vi "CDW_SpecPage.vi"(10 "Spec Page Interface":T2, 11 "MetaDataObj in":refnum<class "MetaDataObj.lvclass">) -> (3 "MetaDataObj out":refnum<class "MetaDataObj.lvclass">)   [LabVIEW 2019, in "NIVS_Consolidated_CDW_MetaDataObj.lvclass"]
uses:
  NIVS_Consolidated_CDW_MetaDataObj.lvclass
  Execution Mode.ctl
  Template Classes/NIVS_Asynchronous/NIVS_Asynchronous.lvclass
  Template Classes/NIVS_Inline HW Interface (Inline-Async)/NIVS_Inline HW Interface (Inline-Async).lvclass
  Template Classes/NIVS_Inline HW Interface/NIVS_Inline HW Interface.lvclass
  Template Classes/NIVS_Inline Model Interface/NIVS_Inline Model Interface.lvclass
  Template Classes/NIVS_Inline Timing and Sync/NIVS_Inline Timing and Sync.lvclass
  Template Classes/NIVS_Asynchronous Timing and Sync/NIVS_Asynchronous Timing and Sync.lvclass
  C:/Program Files (x86)/National Instruments/LabVIEW 2019/resource/dialog/NewProjectWizard/MetaDataObj/MetaDataObj.lvclass
  Template Classes/NIVS_CD Template/NIVS_CD Template.lvclass
  Template Classes/NIVS_PPL_Inline HW Interface (Inline-Async)/NIVS_PPL_Inline HW Interface (Inline-Async).lvclass
  C:/Users/nitest/Git/LabVIEW CD Template Fork/ProjectTemplate/Source/NI VeriStand/Custom Device/Template Classes/NIVS_CD Template/NIVS_CD Template.lvclass
  C:/Users/nitest/Git/LabVIEW CD Template Fork/ProjectTemplate/Source/NI VeriStand/Custom Device/Template Classes/NIVS_Timing and Sync (Abstract)/NIVS_Timing and Sync (Abstract).lvclass
  <resource>/dialog/NewProjectWizard/Spec Page Interface.ctl
  <resource>/dialog/NewProjectWizard/MetaDataObj/MetaDataObj.lvclass
panel:
  in  "PPL Build":bool=TRUE
  in  "Inline-Async":bool=TRUE
  in  "Custom Device Execution Mode":T1(ring)=enum."Inline HW Interface"
  in  "Custom Device Name":string
  in  "Project Root":path
  in  "Maximum Custom Device Instances":u32=1 min=1 max=2474 step=1
  in  "Insert Custom Device in submenu":bool
  in  "Parent Menu Name":string
  in  "Custom Device Extra Page Names":string[](array[string])
  # "Advanced Options"
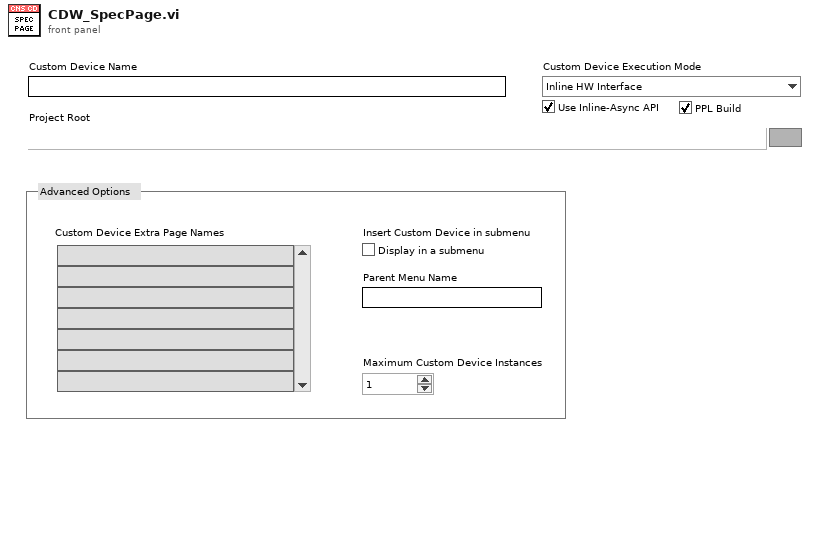
[diagram p1: front panel]
types:
  T1 = enum16{"Asynchronous", "Inline HW Interface", "Inline Model Interface", "Inline Timing and Sync", "Asynchronous Timing and Sync"}
  T2 = typedef "Spec Page Interface.ctl" = cluster{"\"Tab Forward To\" Refnum":refnum<vi>, "\"Tab Backward To\" Refnum":refnum<vi>, "Errors":refnum<user-event>, "Quit":refnum<user-event>}
  T3 = enum8{"Enabled", "Disabled", "Disabled and Grayed Out"}
  T4 = typedef "NIVS_Consolidated_CDW_MetaDataObj.lvclass/Execution Mode.ctl" = enum16{"Asynchronous", "Inline HW Interface", "Inline Model Interface", "Inline Timing and Sync", "Asynchronous Timing and Sync"}
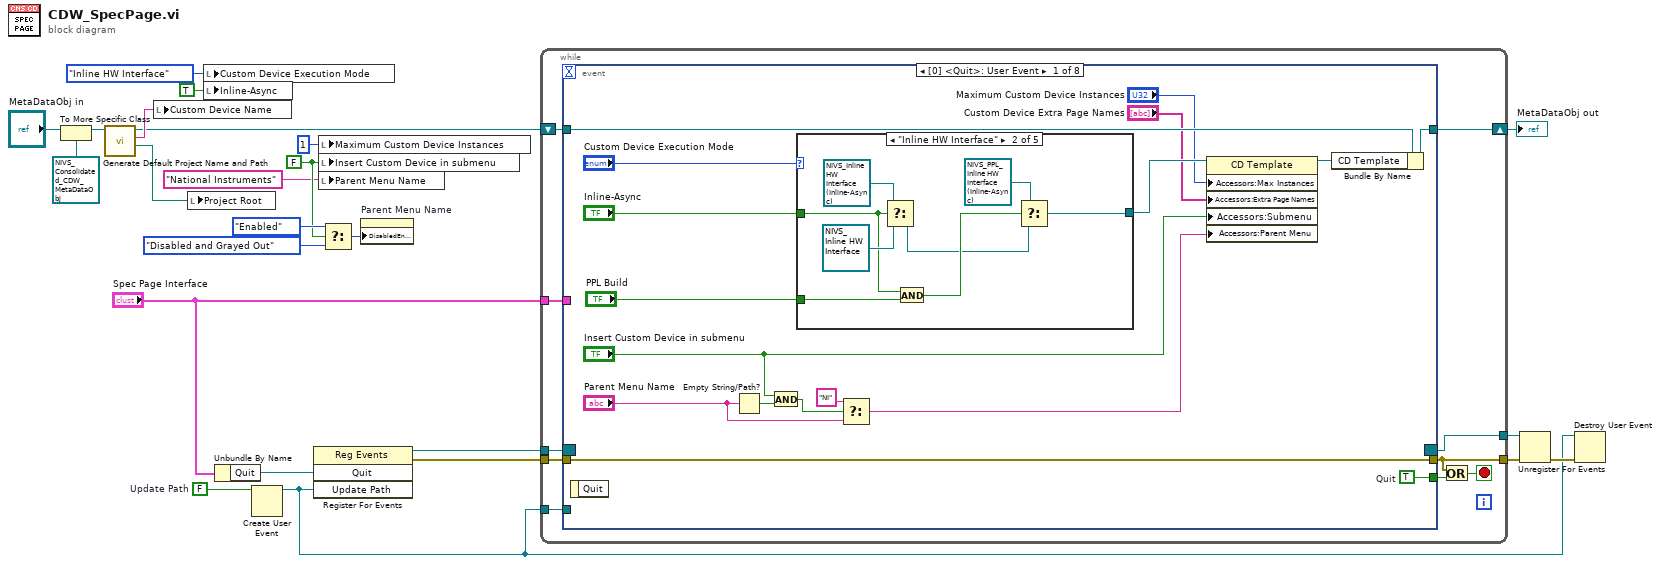
[diagram p0: block diagram]
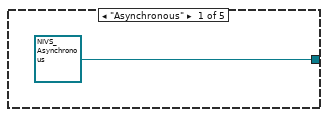
[diagram p2: hidden frame]
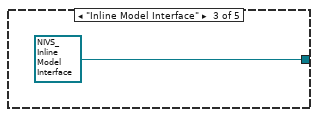
[diagram p3: hidden frame]
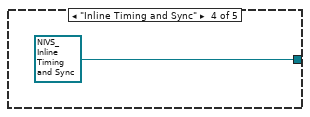
[diagram p4: hidden frame]
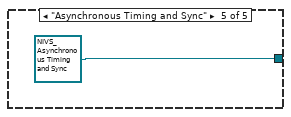
[diagram p5: hidden frame]
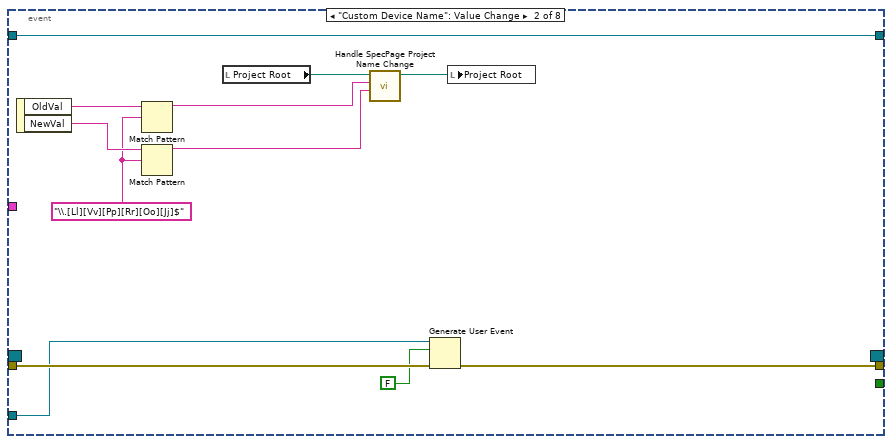
[diagram p6: hidden frame]
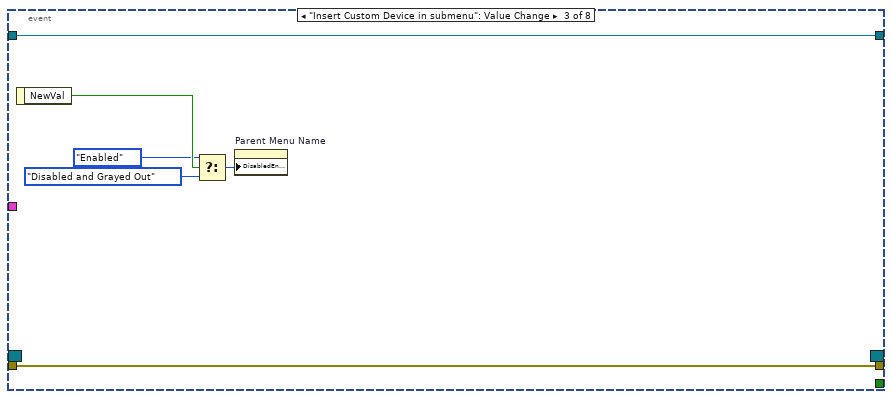
[diagram p7: hidden frame]
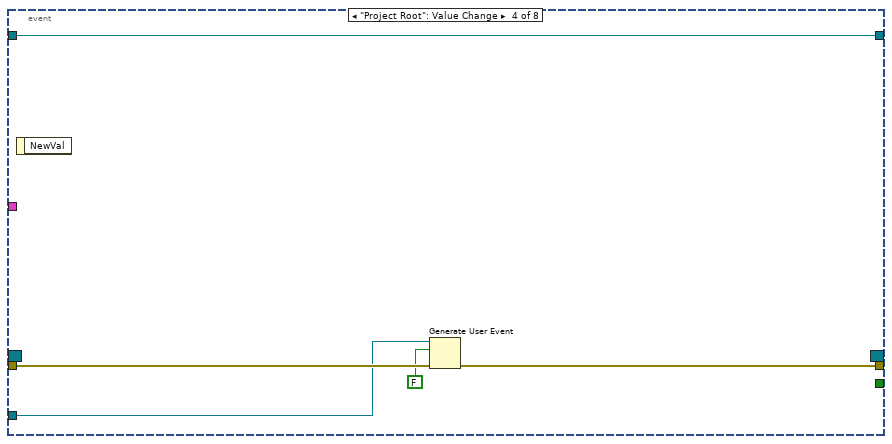
[diagram p8: hidden frame]
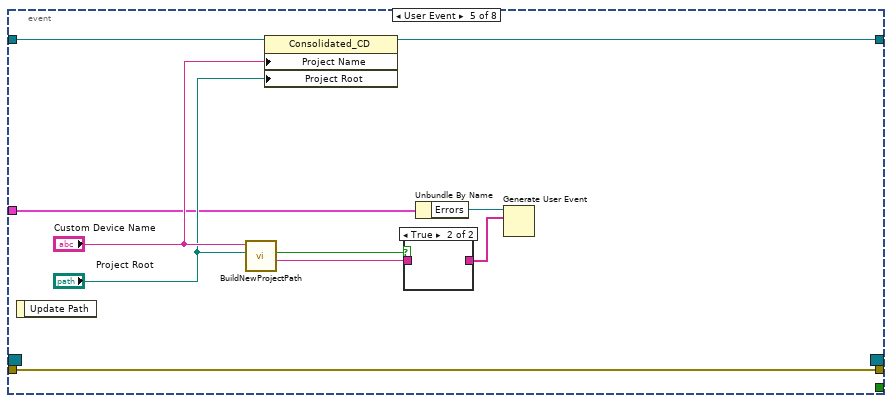
[diagram p9: hidden frame]
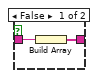
[diagram p10: hidden frame]
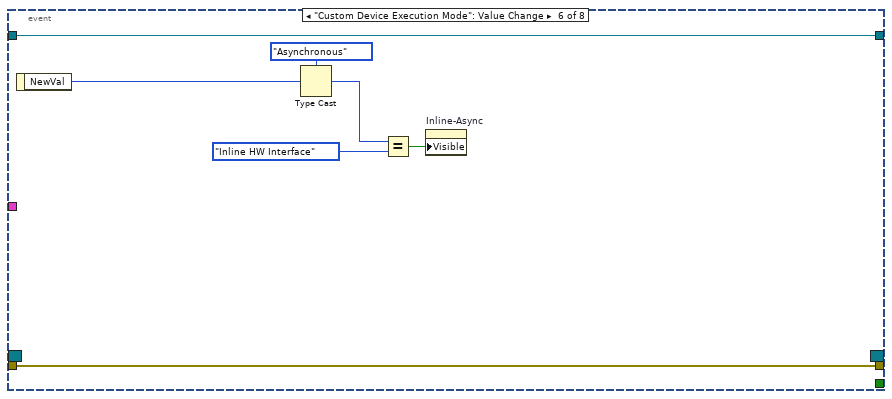
[diagram p11: hidden frame]
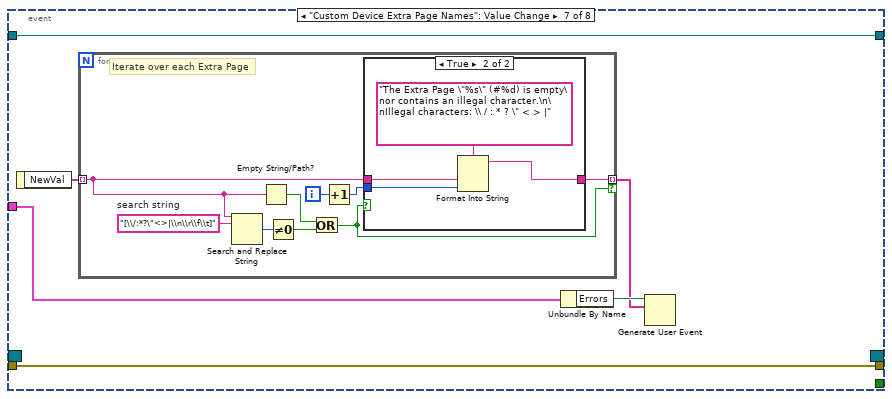
[diagram p12: hidden frame]
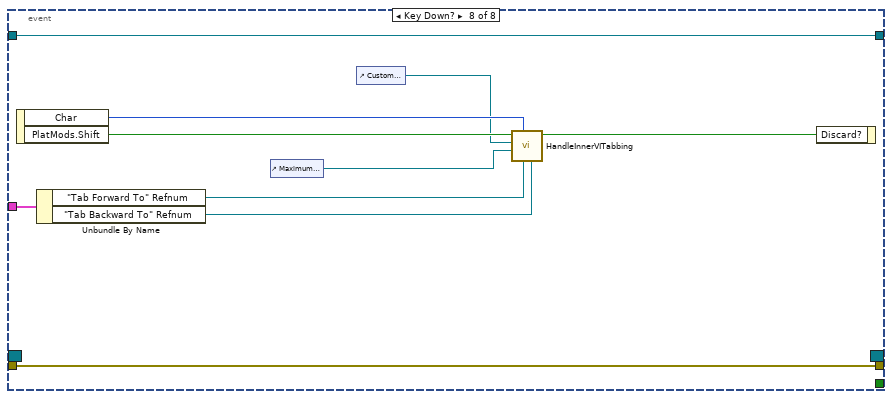
[diagram p14: hidden frame]
diagram:
  w5 = FALSE
  w8 = FALSE  # Update Path
  n1 = To More Specific Class(target class=refnum<class "NIVS_Consolidated_CDW_MetaDataObj.lvclass"> refnum ("Consolidated"), reference="MetaDataObj in") -> (specific class reference=w11:refnum<class "NIVS_Consolidated_CDW_MetaDataObj.lvclass">)  [unwired: 1 in, 1 out]
  n2 = call <resource>:"Generate Default Project Name and Path.vi"("DNL_MetaDataObj in"=w11) -> ("Project Root"=w9:path, "Project Name"=w14:string, "DNL_MetaDataObj out"=w10:refnum<class "NIVS_Consolidated_CDW_MetaDataObj.lvclass">)  [unwired: 8 in]
  n3 = local write "Custom Device Name"(w14) -> ()
  n4 = local write "Project Root"(w9) -> ()
  n5 = local write "Custom Device Execution Mode"(T1."Inline HW Interface" ("Custom Device Execution Mode")) -> ()
  n6 = local write "Inline-Async"(TRUE ("Inline-Async")) -> ()
  n7 = Unbundle By Name("Spec Page Interface") -> ("Quit"=w24:refnum<user-event>)
  n8 = Create User Event(user event datatype=w8) -> (user event=w6:refnum<user-event>)  [unwired: 1 in, 1 out]
  n9 = register-events(w24, w6) -> (reference out=w23:refnum<event-registration>, error out=w19:errorcluster)  [unwired: 2 in]
  n10 = local write "Maximum Custom Device Instances"(u32 1 ("Maximum Custom Device Instances")) -> ()
  n11 = local write "Insert Custom Device in submenu"(w5) -> ()
  n12 = local write "Parent Menu Name"("National Instruments") -> ()
  n13 = Select(t=T3."Enabled" ("Disabled"), s=w5, f=T3."Disabled and Grayed Out") -> (s? t:f=w17:T3)
  n14 = property on="Parent Menu Name" class="Str"("DisabledEnum"=w17) -> ()  [unwired: 2 in, 2 out]
  n15 = while {
    tunnel: "Spec Page Interface" -> [w32]
    shift-right: [w31] -> w20
    shift-left: w10 -> [w30]
    tunnel: w23 -> [w34]
    tunnel: w19 -> [w33]
    tunnel: [w27] -> w21
    tunnel: [w26] -> w13
    tunnel: w6 -> [w25]
    stop <- w29 stop-if-true
    n16 = event shown="[0] <Quit>: User Event" {
      selector: w34 -> [_ _ _ _ _ _ _ _]
      dyn-events: [_ _ _ _ _ _ _ _] -> w26
      timeout: _ -> [_ _ _ _ _ _ _ _]
      tunnel: w32 -> [_ _ _ _ w91 _ w107 w130]
      tunnel: [w51 _ _ _ _ _ _ _] -> w28
      tunnel: [w50 w66 w81 w84 w96 w105 w111 w135] -> w27
      tunnel: w33 -> [w50 w75 w81 w86 w96 w105 w111 w135]
      tunnel: [w48 w74 w80 w85 w94 w104 w109 w134] -> w31
      tunnel: w30 -> [w49 w74 w80 w85 w95 w104 w109 w134]
      tunnel: w25 -> [_ w65 _ w83 _ _ _ _]
      event User Event {
        w51 = TRUE  # Quit
        n17 = event-data() -> ()  [unwired: 1 in, 1 out]
        n18 = Empty String/Path?(string/path="Parent Menu Name") -> (empty?=w46:bool)
        n19 = And(x="Insert Custom Device in submenu", y=w46) -> (x .and. y?=w45:bool)
        n20 = case shown="\"Inline HW Interface\"" "Custom Device Execution Mode" {
          tunnel: "Inline-Async" -> [_ w57 _ _ _]
          tunnel: [refnum<class "NIVS_Asynchronous.lvclass"> refnum ("NIVS_Asynchronous.lvclass") w53 refnum<class "NIVS_Inline Model Interface.lvclass"> refnum ("NIVS_Inline Model Interface.lvclass") refnum<class "NIVS_Inline Timing and Sync.lvclass"> refnum ("NIVS_Inline Timing and Sync.lvclass") refnum<class "NIVS_Asynchronous Timing and Sync.lvclass"> refnum ("NIVS_Asynchronous Timing and Sync.lvclass")] -> w40
          tunnel: "PPL Build" -> [_ w58 _ _ _]
          frame "Asynchronous" {
          }
          frame "Inline HW Interface" {
            n21 = Select(t=refnum<class "NIVS_Inline HW Interface (Inline-Async).lvclass"> refnum ("NIVS_Inline HW Interface (Inline-Async).lvclass"), s=w57, f=refnum<class "NIVS_Inline HW Interface.lvclass"> refnum ("NIVS_Inline HW Interface.lvclass")) -> (s? t:f=w55:refnum<class "NIVS_CD Template.lvclass">)
            n22 = And(x=w57, y=w58) -> (x .and. y?=w56:bool)
            n23 = Select(t=refnum<class "NIVS_PPL_Inline HW Interface (Inline-Async).lvclass"> refnum ("NIVS_PPL_Inline HW Interface (Inline-Async).lvclass"), s=w56, f=w55) -> (s? t:f=w53:refnum<class "NIVS_CD Template.lvclass">)
          }
          frame "Inline Model Interface" {
          }
          frame "Inline Timing and Sync" {
          }
          frame "Asynchronous Timing and Sync" {
          }
        }
        n24 = Select(t="NI", s=w45, f="Parent Menu Name") -> (s? t:f=w36:string)
        n25 = property class="CD Template"(reference=w40, "Accessors:Max Instances"="Maximum Custom Device Instances", "Accessors:Extra Page Names"="Custom Device Extra Page Names", "Accessors:Submenu"="Insert Custom Device in submenu", "Accessors:Parent Menu"=w36) -> (reference out=w41:refnum<class "NIVS_CD Template.lvclass">)  [unwired: 1 in, 1 out]
        n26 = Bundle By Name(cluster=w49, "CD Template"=w41) -> (w48:refnum<class "NIVS_Consolidated_CDW_MetaDataObj.lvclass">)
      }
      event "Custom Device Name": Value Change {
        w71 = "\\.[Ll][Vv][Pp][Rr][Oo][Jj]$"
        n27 = event-data() -> ("OldVal"=w73:string, "NewVal"=w72:string)  [unwired: 1 in]
        n28 = Match Pattern(string=w73, regular expression=w71) -> (before substring=w68:string)  [unwired: 1 in, 3 out]
        n29 = Match Pattern(string=w72, regular expression=w71) -> (before substring=w67:string)  [unwired: 1 in, 3 out]
        n30 = local read "Project Root"() -> (w70:path)
        n31 = call <resource>:"Handle SpecPage Project Name Change.vi"("Project Name New Value"=w67, "Project Name Old Value"=w68, "Project Root in"=w70) -> ("Project Root out"=w69:path)  [unwired: 8 in]
        n32 = Generate User Event(user event=w65, event data cluster=FALSE, error in=w75) -> (error out=w66:errorcluster)  [unwired: 1 in, 1 out]
        n33 = local write "Project Root"(w69) -> ()
      }
      event "Insert Custom Device in submenu": Value Change {
        n34 = event-data() -> ("NewVal"=w79:bool)  [unwired: 1 in]
        n35 = Select(t=T3."Enabled" ("Disabled"), s=w79, f=T3."Disabled and Grayed Out") -> (s? t:f=w76:T3)
        n36 = property on="Parent Menu Name" class="Str"("DisabledEnum"=w76) -> ()  [unwired: 2 in, 2 out]
      }
      event "Project Root": Value Change {
        n37 = event-data() -> ()  [unwired: 1 in, 1 out]
        n38 = Generate User Event(user event=w83, event data cluster=FALSE, error in=w86) -> (error out=w84:errorcluster)  [unwired: 1 in, 1 out]
      }
      event User Event {
        n39 = event-data() -> ()  [unwired: 1 in, 1 out]
        n40 = call <resource>:"BuildNewProjectPath.vi"("Project Root"="Project Root", "Project Name"="Custom Device Name") -> ("Error Message"=w90:string, "Valid?"=w87:bool)  [unwired: 7 in, 1 out]
        n41 = property class="Consolidated_CD"(reference=w95, "Project Name"="Custom Device Name", "Project Root"="Project Root") -> (reference out=w94:refnum<class "NIVS_Consolidated_CDW_MetaDataObj.lvclass">)  [unwired: 1 in, 1 out]
        n42 = case shown="True" w87 {
          tunnel: w90 -> [w98 _]
          tunnel: [w97 _] -> w88
          frame False {
            n43 = Build Array(w98) -> (w97:string[])
          }
          frame True {
          }
        }
        n44 = Unbundle By Name(w91) -> ("Errors"=w89:refnum<user-event>)
        n45 = Generate User Event(user event=w89, event data cluster=w88) -> ()  [unwired: 2 in, 2 out]
      }
      event "Custom Device Execution Mode": Value Change {
        n46 = event-data() -> ("NewVal"=w103:T1)  [unwired: 1 in]
        n47 = Type Cast(type=Execution_Mode."Asynchronous" ("CD Wizard - Internal Data.Common Information.CD Execution Mode"), x=w103) -> (*(type *) &x=w101:T4)
        n48 = Equal?(x=w101, y=Execution_Mode."Inline HW Interface") -> (x = y?=w99:bool)
        n49 = property on="Inline-Async" class="Bool (strict)"("Visible"=w99) -> ()  [unwired: 2 in, 2 out]
      }
      event "Custom Device Extra Page Names": Value Change {
        n50 = event-data() -> ("NewVal"=w110:string[])  [unwired: 1 in]
        n51 = for {
          tunnel: w110 -> [w114] mode=indexing
          tunnel: [w113] -> w106 mode=indexing if=w112
          i -> [w116]
          w120 = "[\\/:*?\"<>|\\n\\r\\f\\t]"  # search string
          # "Iterate over each Extra Page"
          n52 = Search and Replace String(input string=w114, search string=w120) -> (number of replacements=w119:i32)  [unwired: 6 in, 3 out]
          n53 = Empty String/Path?(string/path=w114) -> (empty?=w118:bool)
          n54 = Not Equal To 0?(x=w119) -> (x != 0?=w117:bool)
          n55 = Or(x=w118, y=w117) -> (x .or. y?=w112:bool)
          n56 = Increment(x=w116) -> (x+1=w115:i32)
          n57 = case shown="True" w112 {
            tunnel: w115 -> [_ w123]
            tunnel: w114 -> [w121 w124]
            tunnel: [w121 w122] -> w113
            frame False {
              # "Extra Page Name is OK"
            }
            frame True {
              n58 = Format Into String(format string="The Extra Page \"%s\" (#%d) is empty\nor contains an illegal character.\n\nIllegal characters: \\ / : * ? \" < > |", w124, w123) -> (resulting string=w122:string)  [unwired: 2 in, 1 out]
            }
          }
        }
        n59 = Unbundle By Name(w107) -> ("Errors"=w108:refnum<user-event>)
        n60 = Generate User Event(user event=w108, event data cluster=w106) -> ()  [unwired: 2 in, 2 out]
      }
      event Key Down? {
        n61 = event-data() -> ("Char"=w133:i16, "PlatMods.Shift"=w132:bool)  [unwired: 1 in]
        n62 = Unbundle By Name(w130) -> ("\"Tab Forward To\" Refnum"=w129:refnum<vi>, "\"Tab Backward To\" Refnum"=w128:refnum<vi>)
        n63 = control-ref of="Maximum Custom Device Instances"() -> (w126:refnum<vi>)
        n64 = control-ref of="Custom Device Name"() -> (w127:refnum<vi>)
        n65 = call <resource>:"HandleInnerVITabbing.vi"("Tab Backward To"=w128, "Tab Forward To"=w129, "Char"=w133, "Last Control"=w126, "First Control"=w127, "Shift"=w132) -> ("Discard"=w131:bool)  [unwired: 5 in]
        n66 = event-data("Discard?"=w131) -> ()  [unwired: 1 in, 1 out]
      }
    }
    n67 = Or(x=w27, y=w28) -> (x .or. y?=w29:bool)
  }
  "MetaDataObj out" <- w20
  n68 = Unregister For Events(event registration refnum=w13, error in=w21) -> (error out=w7:errorcluster)
  n69 = Destroy User Event(user event=w6, error in=w7) -> ()  [unwired: 1 out]
